vi "Heart.vi"(8 "error in (no error)":errorcluster, 11 "LINX Resource 3":T1) -> (0 "error out":errorcluster, 1 "LINX Resource 2":T1, 2 "Error Out":errorcluster, 3 "BPM":dbl, 4 "LINX Resource":T1, 5 "Waveform Chart":dbl(graph))   [LabVIEW 2020]
uses:
  <vilib>/MakerHub/LINX/Private/Type Defs/LINX Ref.ctl
  <vilib>/MakerHub/LINX/Private/Type Defs/Platform.ctl
  <vilib>/MakerHub/LINX/Private/Type Defs/Interface.ctl
  <vilib>/MakerHub/LINX/Private/Device/Type Defs/LINX Device Config.ctl
  <vilib>/MakerHub/LINX/Private/Device/Type Defs/TCP Config.ctl
  <vilib>/MakerHub/LINX/Private/Device/Type Defs/Channels.ctl
  heart_rate_monitor_example - Copy/Controls/Detect Threshold Control.ctl
  <vilib>/MakerHub/LINX/Public/Peripherals/Analog/Analog Read 1 Chan.vi
  <vilib>/MakerHub/LINX/Public/Peripherals/Digital/Digital Write 1 Chan.vi
  <vilib>/MakerHub/LINX/Public/Peripherals/Analog/Analog Read N Chans.vi
  <vilib>/MakerHub/LINX/Public/Peripherals/Digital/Digital Write N Chans.vi
  <vilib>/MakerHub/LINX/Private/Local IO/LinxAnalogRead.vi
  <vilib>/MakerHub/LINX/Public/Utilities/Check Channel.vi
  <vilib>/MakerHub/LINX/Private/Local IO/LinxDigitalWrite.vi
  <vilib>/MakerHub/LINX/Private/Utilties/Generate Error.vi
  <vilib>/MakerHub/LINX/LMH-LINX.lvlib
  <vilib>/MakerHub/LINX/Private/Device/Device.lvlib
panel:
  out "Waveform Chart 2":dbl(graph)
  out "Vlu 3":dbl
  out "Vlu 2":dbl
  out "Vlu":dbl
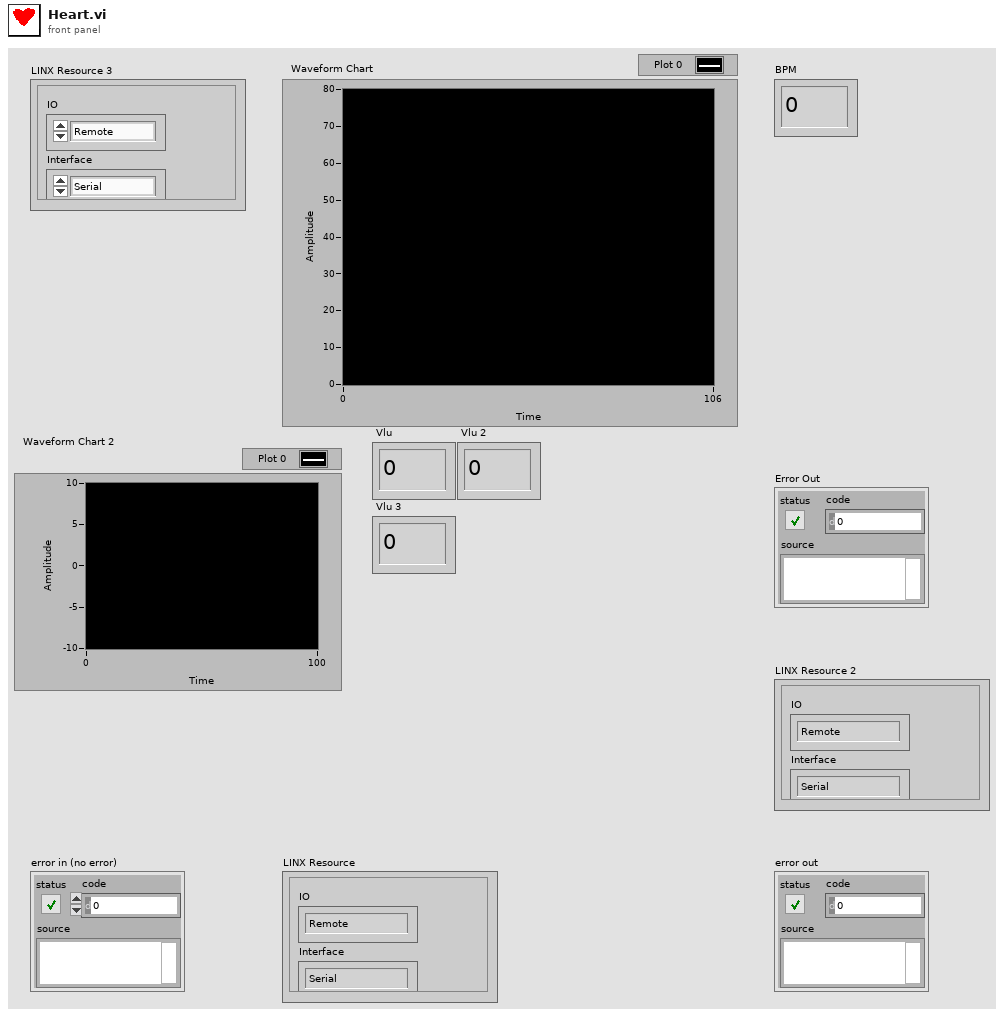
[diagram p1: front panel]
types:
  T1 = typedef "LMH-LINX.lvlib/LINX Ref.ctl" = cluster{"IO":T2, "Interface":T3, "LINX Device Config":T4}
  T2 = typedef "LMH-LINX.lvlib/Platform.ctl" = enum16{"Remote", "Local"}
  T3 = typedef "LMH-LINX.lvlib/Interface.ctl" = enum16{"Serial", "TCP"}
  T4 = typedef "LMH-LINX.lvlib/Device.lvlib/LINX Device Config.ctl" = cluster{"Interface":T3, "COM Port":refnum<visa-resource-name>, "TCP Configuration":T5, "Device Family":u8, "Device ID":u8, "Device Name":string, "TCP Ref":refnum<k5>, "Channels":T6}
  T5 = typedef "LMH-LINX.lvlib/Device.lvlib/TCP Config.ctl" = cluster{"IP Address":string, "Port":u16}
  T6 = typedef "LMH-LINX.lvlib/Channels.ctl" = cluster{"DI":u8[], "DO":u8[], "AI":u8[], "AO":u8[], "PWM":u8[], "QE":u8[], "UART":u8[], "I2C 2":u8[], "SPI":u8[], "CAN":u8[], "Servo":u8[], "AI Ref (V)":dbl, "AI Resolution (Bits)":u8, "AO Ref (V)":dbl, "AO Resolution (Bits)":u8}
  T7 = typedef "Detect Threshold Control.ctl" = enum16{"Get Threshold", "Pulse Found", "Pulse Not Found"}
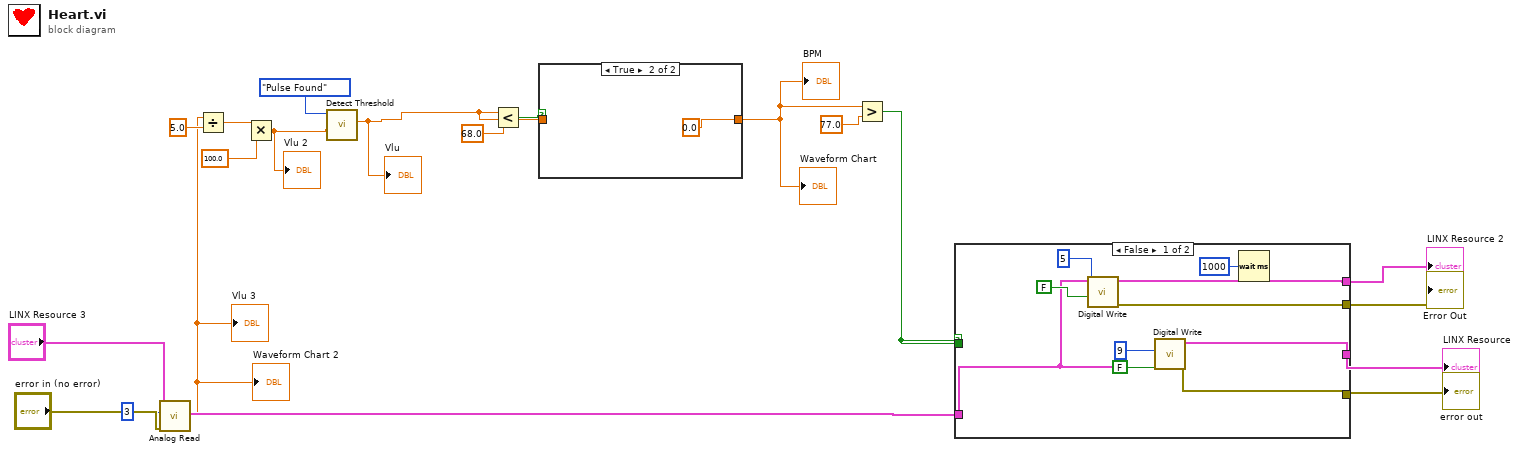
[diagram p0: block diagram]
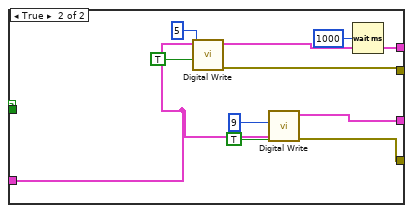
[diagram p2: hidden frame]
diagram:
  n1 = call-poly <vilib>:"Analog Read.vi"("Error In"="error in (no error)", "Analog Channel"=u8 3 ("AI Channel"), "LINX Resource"="LINX Resource 3") -> ("Voltage"=w1:dbl, "LINX Resource"=w14:T1)  [unwired: 5 in, 2 out]
  "Vlu 3" <- w1
  "Waveform Chart 2" <- w1
  n2 = Divide(x=w1, y=5.0) -> (x/y=w6:dbl)
  n3 = Multiply(x=w6, y=100.0) -> (x*y=w2:dbl)
  "Vlu 2" <- w2
  n4 = call "Detect Threshold.vi"("Amplitude"=w2, "Action"=Detect_Threshold_Control."Pulse Found") -> ("Threshold"=w3:dbl)  [unwired: 4 in, 1 out]
  "Vlu" <- w3
  n5 = Less?(x=w3, y=68.0) -> (x < y?=w10:bool)
  n6 = case shown="True" w10 {
    tunnel: [w21 0.0] -> w11
    tunnel: w3 -> [w21 _]
    frame False {
    }
    frame True {
    }
  }
  "Waveform Chart" <- w11
  "BPM" <- w11
  n7 = Greater?(x=w11, y=77.0) -> (0:w13:bool)
  n8 = case shown="False" w13 {
    tunnel: w13 -> [_ _]
    tunnel: w14 -> [w27 w39]
    tunnel: [w25 w40] -> w18
    tunnel: [w26 w38] -> w17
    tunnel: [w24 w34] -> w19
    tunnel: [w23 w33] -> w20
    frame False {
      n9 = call-poly <vilib>:"Digital Write.vi"("Output Value"=FALSE, "DO Channel"=u8 5, "LINX Resource"=w27) -> ("Error Out"=w23:errorcluster, "LINX Resource"=w26:T1)  [unwired: 7 in]
      n10 = call-poly <vilib>:"Digital Write.vi"("Output Value"=FALSE, "DO Channel"=u8 9, "LINX Resource"=w27) -> ("Error Out"=w24:errorcluster, "LINX Resource"=w25:T1)  [unwired: 7 in]
      n11 = Wait (ms)(milliseconds to wait=u32 1000) -> ()  [unwired: 1 out]
    }
    frame True {
      n12 = call-poly <vilib>:"Digital Write.vi"("Output Value"=TRUE, "DO Channel"=u8 5, "LINX Resource"=w39) -> ("Error Out"=w33:errorcluster, "LINX Resource"=w38:T1)  [unwired: 7 in]
      n13 = call-poly <vilib>:"Digital Write.vi"("Output Value"=TRUE, "DO Channel"=u8 9, "LINX Resource"=w39) -> ("Error Out"=w34:errorcluster, "LINX Resource"=w40:T1)  [unwired: 7 in]
      n14 = Wait (ms)(milliseconds to wait=u32 1000) -> ()  [unwired: 1 out]
    }
  }
  "Error Out" <- w20
  "error out" <- w19
  "LINX Resource" <- w18
  "LINX Resource 2" <- w17
